vi "Transfer Group Configuration.Initialize.vi"(8 "error in (no error)":errorcluster, 10 "Transfer Group Configuration cluster":T1={"name"="", "direction"=enum."Tx", "cycle timing"={"priority"=0, "decimation"=1, "offset"=0}, "Transfers"=[], "settings"=[]}, 11 "Transfer Group Configuration in":refnum<class "Transfer Group Configuration.lvclass">) -> (0 "error out":errorcluster, 3 "Transfer Group Configuration":refnum<class "Transfer Group Configuration.lvclass">)   [LabVIEW 2017, in "DSF Core.lvlib" / "Transfer Group Configuration.lvclass"]
uses:
  Transfer Group Configuration.lvclass
  C:/Git/DSF/dsf core/Source/Shared/Classes/Configuration/Configuration.lvclass
  DSF Configuration API/Public/Controls/DSF Engine Transfer Group Configuration.ctl
  DSF Configuration API/Public/Controls/DSF Direction.ctl
  DSF Configuration API/Public/Controls/DSF Timing Info.ctl
  DSF Configuration API/Public/Controls/DSF Engine Transfer Configuration.ctl
  DSF Configuration API/Public/Controls/DSF Byte Order.ctl
  DSF Configuration API/Public/Controls/DSF Engine Channel Configuration.ctl
  DSF Configuration API/Public/Controls/DSF Data Type.ctl
  DSF Configuration API/Public/Controls/DSF Settings Info.ctl
  Configuration/Configuration.lvclass/Configuration.ctl
  Transfer Group Configuration.lvclass/Transfer Group Configuration.ctl
  Transfer/Transfer Configuration.lvclass
  Configuration/Configuration.lvclass
  DSF Core.lvlib
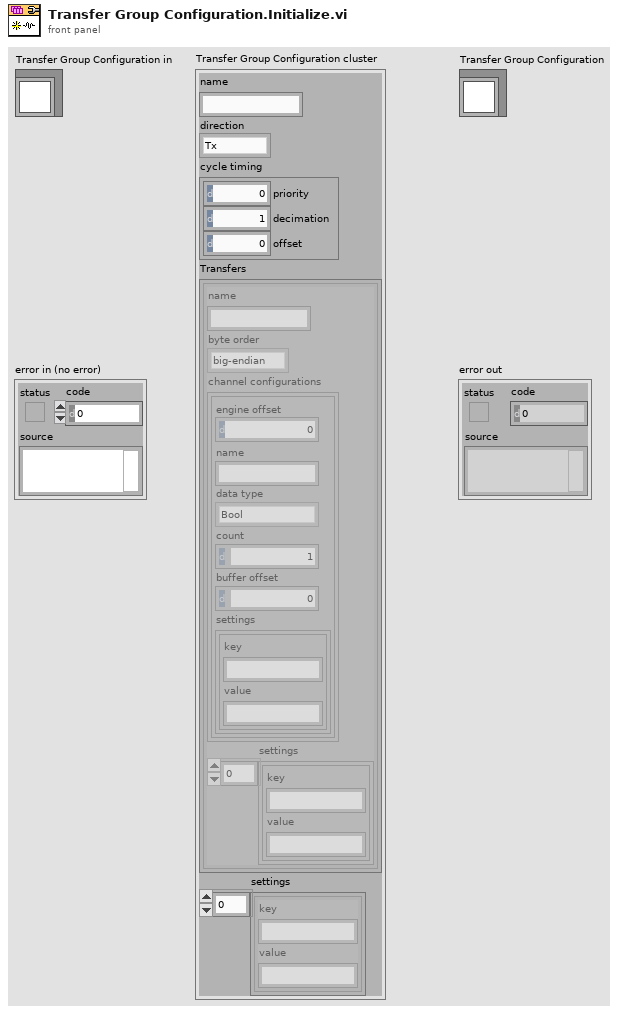
[diagram p1: front panel]
types:
  T1 = typedef "DSF Core.lvlib/DSF Engine Transfer Group Configuration.ctl" = cluster{"name":string, "direction":T2, "cycle timing":T3, "Transfers":T4[], "settings":T8}
  T2 = typedef "DSF Core.lvlib/DSF Direction.ctl" = enum8{"Tx", "Rx"}
  T3 = typedef "DSF Core.lvlib/DSF Timing Info.ctl" = cluster{"priority":u64, "decimation":u64, "offset":u64}
  T4 = typedef "DSF Core.lvlib/DSF Engine Transfer Configuration.ctl" = cluster{"name":string, "byte order":T5, "channel configurations":T6[], "settings":T8}
  T5 = typedef "DSF Core.lvlib/DSF Byte Order.ctl" = enum8{"big-endian", "little-endian"}
  T6 = typedef "DSF Core.lvlib/DSF Engine Channel Configuration.ctl" = cluster{"engine offset":u64, "name":string, "data type":T7, "count":u64, "buffer offset":u64, "settings":T8}
  T7 = typedef "DSF Core.lvlib/DSF Data Type.ctl" = enum8{"Bool", "SGL", "DBL", "I8", "I16", "I32", "I64", "U8", "U16", "U32", "U64"}
  T8 = typedef "DSF Core.lvlib/DSF Settings Info.ctl" = cluster{"key":string, "value":string}[]
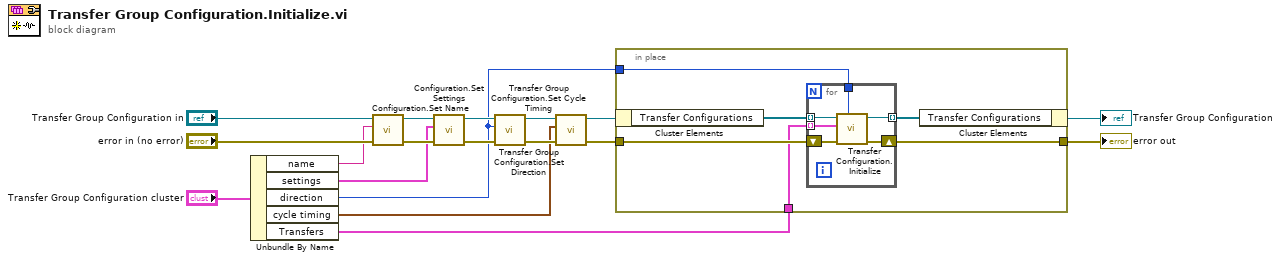
[diagram p0: block diagram]
diagram:
  n1 = Unbundle By Name("Transfer Group Configuration cluster") -> ("name"=w2:string, "settings"=w3:T8, "direction"=w1:T2, "cycle timing"=w10:T3, "Transfers"=w7:T4[])
  n2 = call "Configuration.Set Name.vi"("name"=w2, "Configuration in"="Transfer Group Configuration in") -> ("Configuration out"=w5:refnum<class "Transfer Group Configuration.lvclass">)  [unwired: 9 in]
  n3 = call "Configuration.Set Settings.vi"("settings"=w3, "Configuration in"=w5) -> ("Configuration out"=w4:refnum<class "Transfer Group Configuration.lvclass">)  [unwired: 9 in]
  n4 = call "Transfer Group Configuration.Set Direction.vi"("direction"=w1, "Transfer Group Configuration in"=w4) -> ("Transfer Group Configuration out"=w13:refnum<class "Transfer Group Configuration.lvclass">)  [unwired: 9 in]
  n5 = call "Transfer Group Configuration.Set Cycle Timing.vi"("cycle timing"=w10, "Transfer Group Configuration in"=w13) -> ("Transfer Group Configuration out"=w12:refnum<class "Transfer Group Configuration.lvclass">)  [unwired: 9 in]
  n6 = in-place {
    in-place-border: "error in (no error)" -> [w18]
    in-place-border: [w17] -> w9
    in-place-border: w7 -> [w16]
    in-place-border: w1 -> [w15]
    n7 = in-place-cluster #1(w12) -> ("Transfer Configurations"=w20:refnum<class "Transfer Configuration.lvclass">[])
    n8 = for {
      tunnel: w20 -> [w26] mode=indexing
      tunnel: [w25] -> w19 mode=indexing
      shift-right: [w24] -> w17
      shift-left: w18 -> [w23]
      tunnel: w16 -> [w22] mode=indexing
      tunnel: w15 -> [w21]
      n9 = call-dynamic "Transfer Configuration.Initialize.vi"("direction"=w21, "error in (no error)"=w23, "Transfer Configuration cluster"=w22, "Transfer Configuration in"=w26) -> ("error out"=w24:errorcluster, "Transfer Configuration out"=w25:refnum<class "Transfer Configuration.lvclass">)  [unwired: 6 in]
    }
    n10 = in-place-cluster #1("Transfer Configurations"=w19) -> (→"Transfer Group Configuration":refnum<class "Transfer Group Configuration.lvclass">)
  }
  "error out" <- w9
